vi "Robot Fail.vi"() -> ()   [LabVIEW 2014]
panel:
  out "Failures":T1
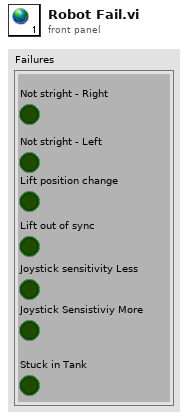
[diagram p1: front panel]
types:
  T1 = cluster{"Not stright - Right":bool, "Not stright - Left":bool, "Lift position change":bool, "Lift out of sync":bool, "Joystick sensitivity Less":bool, "Stuck in Tank":bool, "Joystick Sensistiviy More":bool}
diagram:
